vi "2D_array_from_string.vi"(1 "String Name":string, 2 "Show Dialog?":bool, 3 "Input string":string, 4 "Array title":string) -> (0 "2D data array":dbl[][](array[numeric]) format="%.2f")   [LabVIEW 2010]
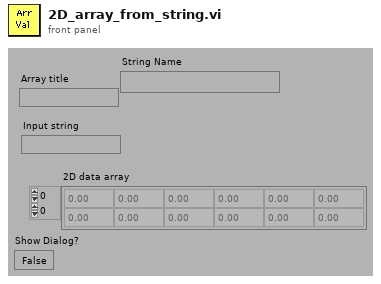
[diagram p1: front panel]
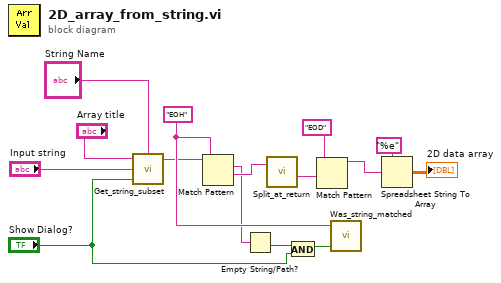
[diagram p0: block diagram]
diagram:
  w9 = "EOH"
  n1 = call "Get_string_subset.vi"("String Name"="String Name", "Show Dialog?"="Show Dialog?", "String to split"="Input string", "File Label"="Array title") -> ("Output string"=w8:string)  [unwired: 1 out]
  n2 = Match Pattern(string=w8, regular expression=w9) -> (match substring=w5:string, after substring=w15:string)  [unwired: 3 out]
  n3 = Empty String/Path?(string/path=w5) -> (empty?=w4:bool)
  n4 = call "Split_at_return.vi"("String"=w15) -> ("after substring"=w14:string)  [unwired: 1 in, 3 out]
  n5 = And(x=w4, y="Show Dialog?") -> (x .and. y?=w2:bool)
  n6 = Match Pattern(string=w14, regular expression="EOD") -> (before substring=w12:string)  [unwired: 4 out]
  n7 = call "Was_string_matched.vi"("Match Error"=w2, "Variable name"=w9) -> ()  [unwired: 1 in]
  n8 = Spreadsheet String To Array(format string="%e", spreadsheet string=w12) -> (array=→"2D data array":dbl[][])  [unwired: 2 out]
